vi "Host-ItchParser-TestHarness.vi"() -> ()   [LabVIEW 2016]
uses:
  <vilib>/rvi/interface/RandomDataEmulation/nirviRandomDataOpen.vi
  <vilib>/rvi/interface/RandomDataEmulation/nirviRandomDataDMAMethods.vi
  <vilib>/rvi/interface/RandomDataEmulation/nirviRandomDataClose.vi
  <vilib>/rvi/interface/nirviOpenFPGA/nirviOpenFPGA.xnode
  ItchParser-TestHarness-Typedef.ctl
  Fpga/Tests/Fpga-ItchParser-TestHarness.vi
  <vilib>/rvi/interface/nirviMethod/nirviMethod.xnode
  <vilib>/rvi/interface/nirviCloseFPGA/nirviCloseFPGA.xnode
panel:
  out "OrderBook Operations":T1(array[cluster])
  out "error out":errorcluster
  in  "file path (use dialog)":path
  in  "error in":errorcluster
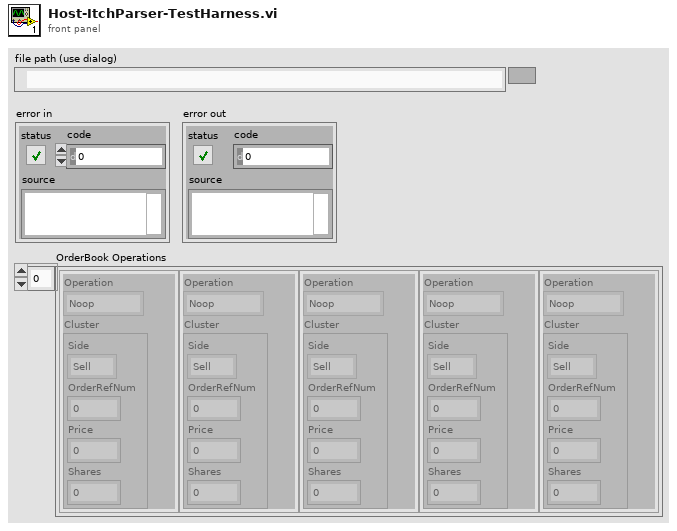
[diagram p1: front panel]
types:
  T1 = cluster{"Operation":enum16{"Noop", "GetAll", "AddOrder", "DeleteOrder"}, "Cluster":cluster{"Side":enum16{"Sell", "Buy"}, "OrderRefNum":u64, "Price":u32, "Shares":u32}}[]
  T2 = typedef "ItchParser-TestHarness-Typedef.ctl" = refnum<k20>
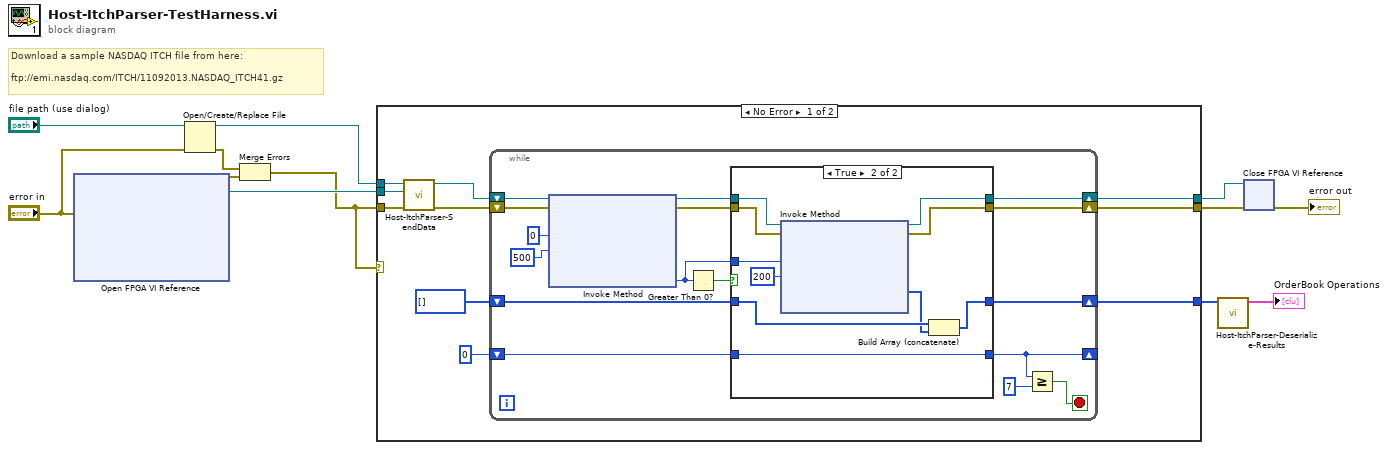
[diagram p0: block diagram]
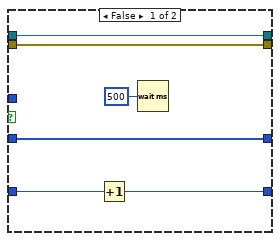
[diagram p2: hidden frame]
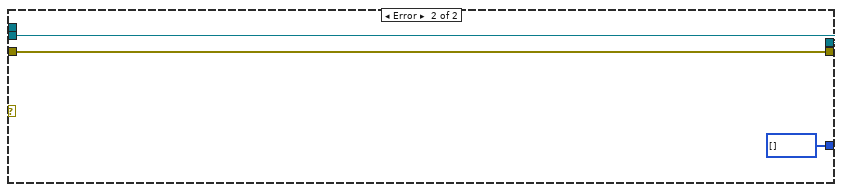
[diagram p3: hidden frame]
diagram:
  # "Download a sample NASDAQ ITCH file from here:\n\nftp://emi.nasdaq.com/ITCH/11092013.NASDAQ_ITCH41.gz"
  n1 = xnode "Open FPGA VI Reference"("error in"="error in") -> ("FPGA VI Reference Out"=w12:T2, "error out"=w7:errorcluster)  [unwired: 1 in]
  n2 = Open/Create/Replace File(file path (use dialog)="file path (use dialog)", error in="error in") -> (refnum out=w10:refnum<file>, error out=w8:errorcluster)  [unwired: 4 in, 1 out]
  n3 = Merge Errors(w8, w7) -> (w6:errorcluster)
  n4 = case shown="No Error" w6 {
    tunnel: w12 -> [w22 w56]
    tunnel: [w17 w57] -> w4
    tunnel: w10 -> [w19 _]
    tunnel: w6 -> [w18 w57]
    tunnel: [w16 w56] -> w3
    tunnel: [w13 u64[] [] ("Data 2")] -> w2
    frame No Error {
      n5 = call "Host-ItchParser-SendData.vi"("error in\n(no error)"=w18, "FPGA VI Reference Out 3"=w22, "Byte Stream\nFile in"=w19) -> ("error out"=w20:errorcluster, "FPGA VI Reference Out 2"=w21:T2)  [unwired: 7 in]
      n6 = while {
        shift-right: [w27] -> w13
        shift-left: u64[] [] ("Data 2") -> [w28]
        shift-right: [w30] -> w16
        shift-left: w21 -> [w38]
        shift-right: [w29] -> w17
        shift-left: w20 -> [w31]
        shift-right: [w25] -> _
        shift-left: 0 -> [w26]
        stop <- w23 stop-if-true
        n7 = xnode "Invoke Method"("FPGA VI Reference In"=w38, "error in"=w31, "Number of Elements"=u32 0, "Timeout (ms)"=500) -> ("FPGA VI Reference Out"=w33:T2, "error out"=w32:errorcluster, "Elements Remaining"=w34:u32)  [unwired: 1 out]
        n8 = Greater Than 0?(x=w34) -> (x > 0?=w35:bool)
        n9 = case shown="True" w35 {
          tunnel: w34 -> [_ w54]
          tunnel: w33 -> [w44 w52]
          tunnel: w32 -> [w43 w51]
          tunnel: [w44 w50] -> w30
          tunnel: [w43 w49] -> w29
          tunnel: w28 -> [w42 w48]
          tunnel: [w42 w46] -> w27
          tunnel: [w40 w45] -> w25
          tunnel: w26 -> [w41 w45]
          frame False {
            n10 = Increment(x=w41) -> (x+1=w40:i32)
            n11 = Wait (ms)(milliseconds to wait=u32 500) -> ()  [unwired: 1 out]
          }
          frame True {
            n12 = xnode "Invoke Method"("FPGA VI Reference In"=w52, "error in"=w51, "Number of Elements"=w54, "Timeout (ms)"=200) -> ("FPGA VI Reference Out"=w50:T2, "error out"=w49:errorcluster, "Data"=w47:u64[])  [unwired: 1 out]
            n13 = Build Array (concatenate)(w48, w47) -> (w46:u64[])
          }
        }
        n14 = Greater Or Equal?(x=w25, y=7) -> (x >= y?=w23:bool)
      }
    }
    frame Error {
    }
  }
  n15 = call "Host-ItchParser-Deserialize-Results.vi"("Data in"=w2) -> ("Array"=→"OrderBook Operations":T1)  [unwired: 10 in]
  n16 = xnode "Close FPGA VI Reference"("FPGA VI Reference In"=w3, "error in"=w4) -> ("error out"=→"error out":errorcluster)
